vi "Node - Close.vi"(8 "error in (no error)":errorcluster, 11 "Node Data In":T1) -> (0 "error out":errorcluster)   [LabVIEW 2016, in "PXImc Router.lvlib"]
uses:
  PXImc Router.lvlib
  Controls/Node Data.ctl
  <vilib>/NI Veristand/VeriStand Data/Byte Buffer/Byte Buffer.lvclass
  Controls/Node/Node - PXImc Parameters.ctl
  Controls/Node/Node - Writer Data.ctl
  Controls/Node/Node Ch Properties.ctl
  Controls/Data Type.ctl
  Controls/Node/Node - Readers Data.ctl
  Controls/Node/Node - Reader Data.ctl
  <vilib>/NI Veristand/VeriStand Data/Byte Buffer/Byte Buffer.lvclass/Byte Buffer.ctl
  <vilib>/NI Veristand/VeriStand Data/Byte Buffer/Byte Buffer.Get Buffer Pointer.vi
  <vilib>/NI Veristand/VeriStand Data/Byte Buffer/Byte Buffer.Get Buffer Size.vi
  <vilib>/NI Veristand/VeriStand Data/Pointer Operations/Pointer.Dispose.vi
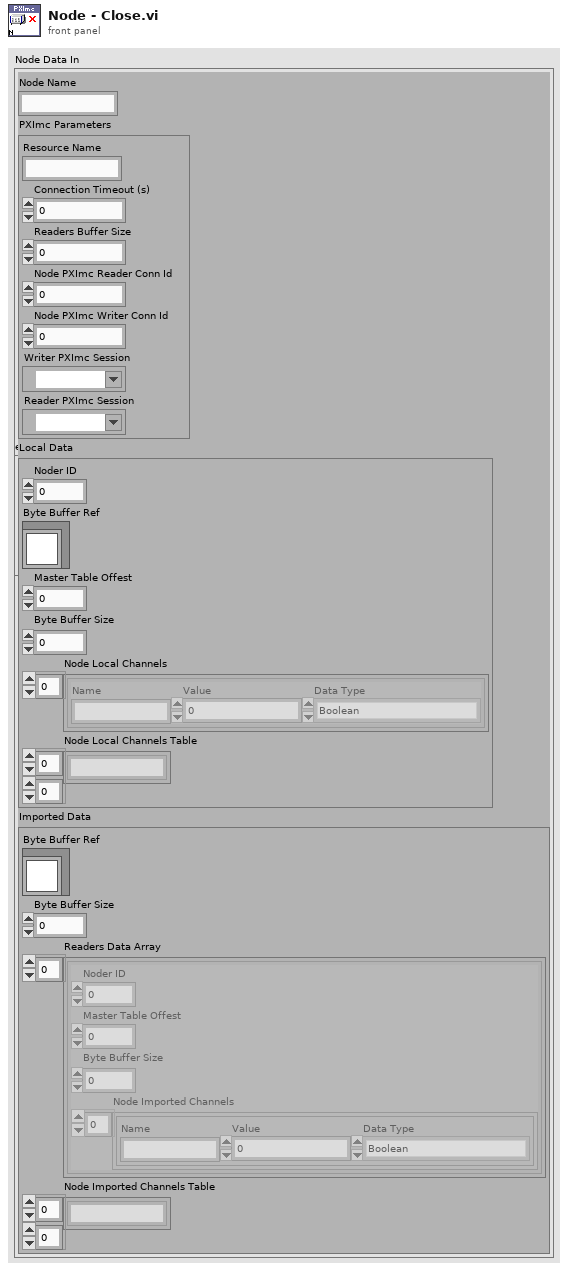
[diagram p1: front panel]
types:
  T1 = typedef "PXImc Router.lvlib/Node Data.ctl" = cluster{"Node Name":string, "PXImc Parameters":T2, "Local Data":T3, "Imported Data":T6}
  T2 = typedef "PXImc Router.lvlib/Node - PXImc Parameters.ctl" = cluster{"Resource Name":string, "Connection Timeout (s)":dbl, "Readers Buffer Size":u64, "Node PXImc Reader Conn Id":u16, "Node PXImc Writer Conn Id":u16, "Writer PXImc Session":refnum<k21>, "Reader PXImc Session":refnum<k21>}
  T3 = typedef "PXImc Router.lvlib/Node - Writer Data.ctl" = cluster{"Noder ID":u32, "Byte Buffer Ref":refnum<class "Byte Buffer.lvclass">, "Master Table Offest":u32, "Byte Buffer Size":u32, "Node Local Channels":T4[], "Node Local Channels Table":string[][]}
  T4 = typedef "PXImc Router.lvlib/Node Ch Properties.ctl" = cluster{"Name":string, "Value":dbl, "Data Type":T5}
  T5 = typedef "PXImc Router.lvlib/Data Type.ctl" = enum16{"Boolean", "SGL", "DBL", "I8", "I16", "I32", "I64", "U8", "U16", "U32", "U64"}
  T6 = typedef "PXImc Router.lvlib/Node - Readers Data.ctl" = cluster{"Byte Buffer Ref":refnum<class "Byte Buffer.lvclass">, "Byte Buffer Size":u64, "Readers Data Array":T7[], "Node Imported Channels Table":string[][]}
  T7 = typedef "PXImc Router.lvlib/Node - Reader Data.ctl" = cluster{"Noder ID":u32, "Master Table Offest":u32, "Byte Buffer Size":u64, "Node Imported Channels":T4[]}
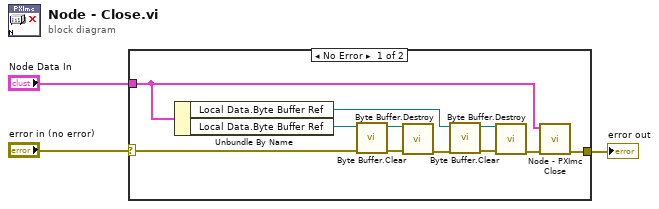
[diagram p0: block diagram]
diagram:
  n1 = case shown="No Error" "error in (no error)" {
    selector: "error in (no error)" -> [w10 w15]
    tunnel: [w7 w15] -> w3
    tunnel: "Node Data In" -> [w14 _]
    frame No Error {
      n2 = Unbundle By Name(w14) -> ("Local Data.Byte Buffer Ref"=w11:refnum<class "Byte Buffer.lvclass">, "Local Data.Byte Buffer Ref"=w4:refnum<class "Byte Buffer.lvclass">)
      n3 = call <vilib>:"Byte Buffer.Clear.vi"("error in (no error)"=w10, "Byte Buffer in"=w4) -> ("error out"=w6:errorcluster, "Byte Buffer out"=w5:refnum<class "Byte Buffer.lvclass">)  [unwired: 8 in]
      n4 = call <vilib>:"Byte Buffer.Destroy.vi"("error in (no error)"=w6, "Byte Buffer in"=w5) -> ("error out"=w9:errorcluster)  [unwired: 9 in]
      n5 = call <vilib>:"Byte Buffer.Clear.vi"("error in (no error)"=w9, "Byte Buffer in"=w11) -> ("error out"=w13:errorcluster, "Byte Buffer out"=w12:refnum<class "Byte Buffer.lvclass">)  [unwired: 8 in]
      n6 = call <vilib>:"Byte Buffer.Destroy.vi"("error in (no error)"=w13, "Byte Buffer in"=w12) -> ("error out"=w8:errorcluster)  [unwired: 9 in]
      n7 = call "Node - PXImc Close.vi"("error in (no error)"=w8, "Node Data In"=w14) -> ("error out"=w7:errorcluster)  [unwired: 8 in, 1 out]
    }
    frame Error {
    }
  }
  "error out" <- w3
